vi "getSampling.vi"(8 "error in (no error)":errorcluster, 11 "Instrument.LockinAPI in":refnum<class "Instrument.LockinAPI.lvclass">) -> (0 "error out":errorcluster, 2 "sampling":T1={"Fs"=204789.0, "#s"=15753}, 3 "Instrument.LockinAPI out":refnum<class "Instrument.LockinAPI.lvclass">)   [LabVIEW 2019, in "Instrument.LockinAPI.lvclass"]
doc: "API to get the AI waveforms.\n\nIf address=\"\", this API reads from localhost\nIf address is remote lockin, you need to add this computer to allowed whitelist on the lockin computer you are trying to access."
uses:
  Instrument.LockinAPI.lvclass
  Typedefs/API/LockinAPI.Sampling.Sampling--Cluster.ctl
  C:/Users/patrick/Documents/GitHub/Instrument-Framework/lvsrc/Instrument/Instrument.lvclass
  Typedefs/API/LockinAPI.Commands--Enum.ctl
  20b6b077-1261-454d-9919-a4eeb7fdd162.vi
  20b6b077-1261-454d-9919-a4eeb7fdd162.vi/aa303d38-ff67-4775-a95d-5ce59cff89c3.vi
  20b6b077-1261-454d-9919-a4eeb7fdd162.vi/aa303d38-ff67-4775-a95d-5ce59cff89c3.vi/794ff5f0-457e-45cb-8088-81d17b4e8c64.vi
  20b6b077-1261-454d-9919-a4eeb7fdd162.vi/aa303d38-ff67-4775-a95d-5ce59cff89c3.vi/6d1cfe07-0388-4bc8-8682-99e45dd3adfe.vi
  20b6b077-1261-454d-9919-a4eeb7fdd162.vi/aa303d38-ff67-4775-a95d-5ce59cff89c3.vi/659a61a6-405f-440b-8c68-093fc753e2c8.vi
  <vilib>/JDP Science/JSONtext/Make JSON Array.vi
  20b6b077-1261-454d-9919-a4eeb7fdd162.vi/aa303d38-ff67-4775-a95d-5ce59cff89c3.vi/6d1cfe07-0388-4bc8-8682-99e45dd3adfe.vi/6ce0be2e-324e-4b75-8219-52f32e2984c2.vi
  20b6b077-1261-454d-9919-a4eeb7fdd162.vi/aa303d38-ff67-4775-a95d-5ce59cff89c3.vi/659a61a6-405f-440b-8c68-093fc753e2c8.vi/c1d2b985-18e3-4e1b-853f-e80a6cc34949.vi
  20b6b077-1261-454d-9919-a4eeb7fdd162.vi/aa303d38-ff67-4775-a95d-5ce59cff89c3.vi/659a61a6-405f-440b-8c68-093fc753e2c8.vi/88dbbb25-94da-49ef-8b4f-dc23b0d307de.vi
  Instrument/API/Enum to String.vi
  Instrument/Private/Get RC Connection Status.vi
  <vilib>/JDP Science/JSONtext/Variant to JSON Text.vi
  <vilib>/JDP Science/JSONtext/support/Format JSON Array Text.vi
  Instrument/API/Send and Receive.vi
  <vilib>/JDP Science/JSONtext/JSON text to Variant.vi
  <vilib>/Utility/Data Type/Get Type Information.vi
  <vilib>/JDP Science/JSONtext/LVClass Serializer/JSONtext LVClass Serializer.lvclass
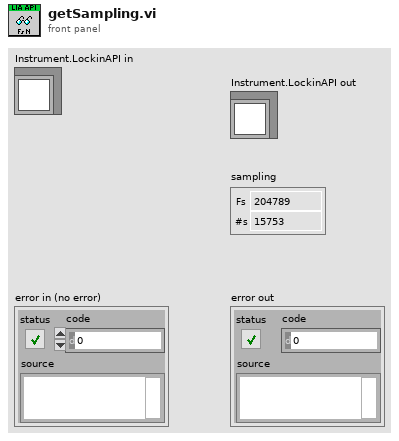
[diagram p1: front panel]
types:
  T1 = typedef "Instrument.LockinAPI.lvclass/LockinAPI.Sampling.Sampling--Cluster.ctl" = cluster{"Fs":dbl, "#s":i32}
  T2 = typedef "Instrument.LockinAPI.lvclass/LockinAPI.Commands--Enum.ctl" = enum16{"setAI", "setAO", "setAO_Amplitude", "setAO_DC", "setAO_Frequency", "setAO_Phase", "setAO_Function", "setAO_I+", "setREF", "setREF_Frequency", "setREF_Phase", "setREF_TC", "setREF_Roll-Off", "setDAQ", "setSampling", "setOffset", "setState", "getState", "getAO", "getAI", "getResults", "getSampling", "getAOconfig", "getREFconfig", "setInputGain", "setOutputGain", "getInputGain", "getOutputGain", "setSamplingMode", "getSamplingMode", "setSweep", "setSweepTime", "setSweepTable", "getStatus", "getSweepResults", "getSweepWaveforms", "startSweep", "stopSweep", "setAUX", "getAUX"}
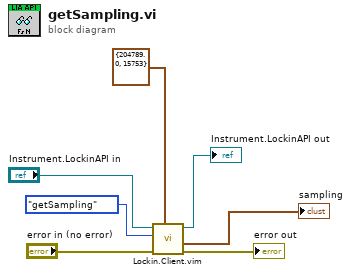
[diagram p0: block diagram]
diagram:
  n1 = call "Lockin.Client.vim"("Data Out type"=T1 {"Fs"=204789.0, "#s"=15753} ("sampling"), "error in (no error)"="error in (no error)", "Command"=LockinAPI.Commands--Enum."getSampling", "Instrument.LockinAPI in"="Instrument.LockinAPI in") -> ("error out"=→"error out":errorcluster, "Data out"=→"sampling":T1, "Instrument.LockinAPI out"=→"Instrument.LockinAPI out":refnum<class "Instrument.LockinAPI.lvclass">)  [unwired: 5 in]
